vi "SaveWWWImages2.vi"(7 "Tab charts":refnum<vi>, 9 "Image Data 2":T1, 10 "Destination":path, 11 "VI in":refnum<vi>) -> ()   [LabVIEW 2017]
uses:
  Web Imge control.ctl
panel:
  out "Write Imegtime":u32
  out "get Imegtime":u32
  out "Time":u32
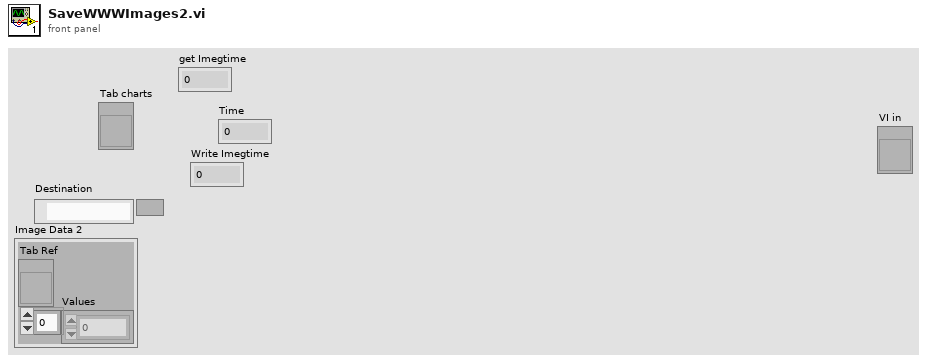
[diagram p1: front panel]
types:
  T1 = typedef "Web Imge control.ctl" = cluster{"Tab Ref":refnum<vi>, "Values":i32[]}
  T2 = typedef "imagedata.ctl" = cluster{"image type":i32, "image depth":i32, "image":u8[], "mask":u8[], "colors":u32[], "Rectangle":cluster{"left":i16, "top":i16, "right":i16, "bottom":i16}}
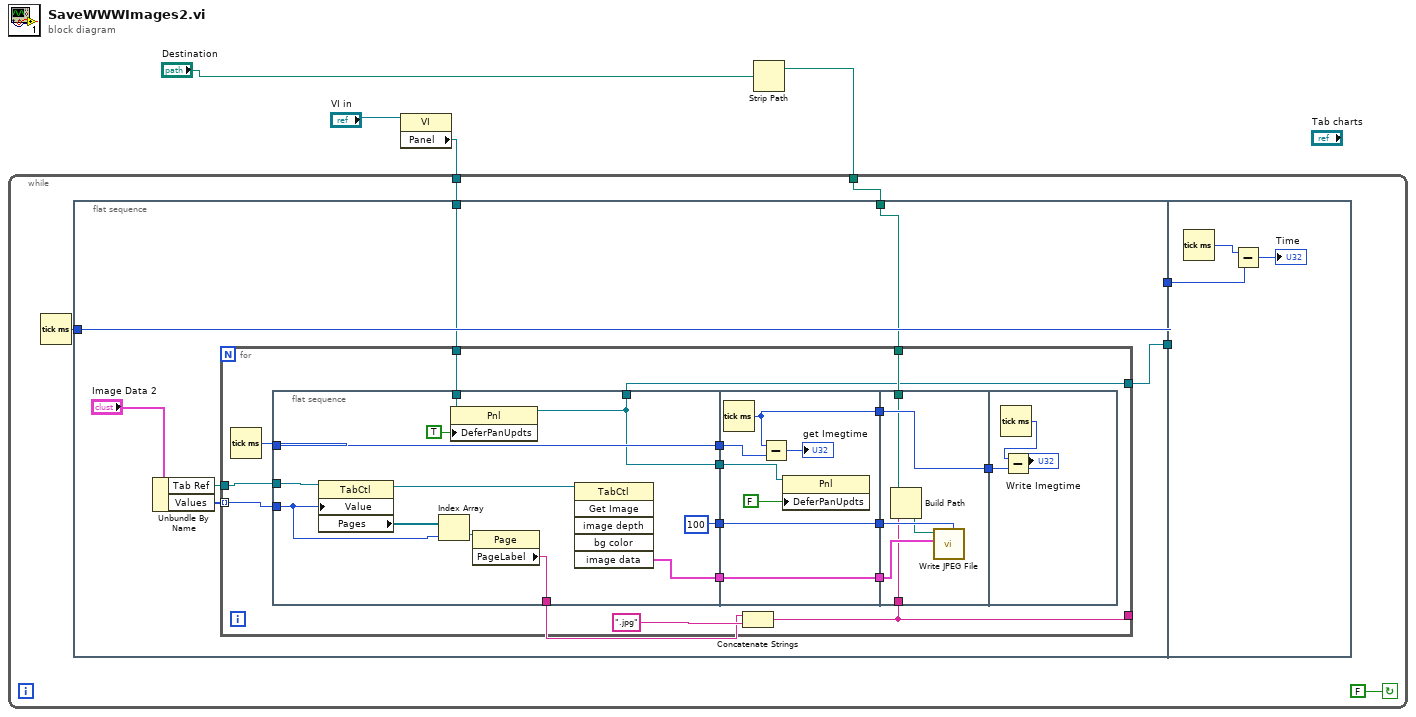
[diagram p0: block diagram]
diagram:
  n1 = property class="VI"(reference="VI in") -> ("Panel"=w1:refnum<vi>)  [unwired: 1 in, 2 out]
  n2 = Strip Path(path="Destination") -> (stripped path=w2:path)  [unwired: 1 out]
  n3 = while {
    tunnel: w2 -> [w6]
    tunnel: w1 -> [w5]
    stop <- FALSE continue-if-true
    n4 = Tick Count (ms)() -> (millisecond timer value=w8:u32)
    n5 = flat-sequence {
      tunnel: [w11] -> w10
      tunnel: [w17] -> w9
      tunnel: w8 -> [w17]
      tunnel: w6 -> [w13]
      tunnel: w5 -> [w12]
      tunnel: w10 -> [_]
      tunnel: w9 -> [w64]
      frame #0 {
        n6 = Unbundle By Name("Image Data 2") -> ("Tab Ref"=w16:refnum<vi>, "Values"=w15:i32[])
        n7 = for {
          tunnel: [w21] -> _
          tunnel: w16 -> [w25]
          tunnel: w15 -> [w24] mode=indexing
          tunnel: w13 -> [w22]
          tunnel: w12 -> [w20]
          tunnel: [w19] -> w11
          n8 = Tick Count (ms)() -> (millisecond timer value=w26:u32)
          n9 = flat-sequence {
            tunnel: w25 -> [w46]
            tunnel: [w44] -> w34
            tunnel: [100 ("quality (80)")] -> w33
            tunnel: [w42] -> w32
            tunnel: w26 -> [w42]
            tunnel: w24 -> [w41]
            tunnel: [w38] -> w23
            tunnel: w20 -> [w37]
            tunnel: [w35] -> w19
            tunnel: [w35] -> w18
            tunnel: w34 -> [w53]
            tunnel: [w53] -> w31
            tunnel: w33 -> [w52]
            tunnel: [w52] -> w30
            tunnel: w32 -> [w51]
            tunnel: [w49] -> w29
            tunnel: w18 -> [w47]
            tunnel: w31 -> [w58]
            tunnel: w30 -> [w59]
            tunnel: w29 -> [w57]
            tunnel: [w57] -> w28
            tunnel: w22 -> [w56]
            tunnel: w21 -> [w54]
            tunnel: w28 -> [w60]
            frame #0 {
              n10 = property class="TabCtl"(reference=w46, "Value"=w41) -> (reference out=w45:refnum<vi>, "Pages"=w40:refnum<vi>[])  [unwired: 1 in, 1 out]
              n11 = Index Array(array=w40, index=w41) -> (element=w39:refnum<vi>)
              n12 = property class="Pnl"(reference=w37, "DeferPanUpdts"=TRUE ("Defer Panel Updates")) -> (reference out=w35:refnum<vi>)  [unwired: 1 in, 1 out]
              n13 = property class="Page"(reference=w39) -> ("PageLabel"=w38:string)  [unwired: 1 in, 2 out]
              n14 = invoke class="TabCtl" method="Get Image"(reference=w45) -> ("image data"=w44:T2)  [unwired: 5 in, 5 out]
            }
            frame #1 {
              n15 = Tick Count (ms)() -> (millisecond timer value=w49:u32)
              n16 = Subtract(x=w49, y=w51) -> (x-y=→"get Imegtime":u32)
              n17 = property class="Pnl"(reference=w47, "DeferPanUpdts"=FALSE ("Defer Panel Updates")) -> ()  [unwired: 1 in, 2 out]
            }
            frame #2 {
              n18 = Build Path(base path=w56, name or relative path=w54) -> (appended path=w55:path)
              n19 = call <vilib>:"Write JPEG File.vi"("quality (80)"=w59, "image data"=w58, "path to JPEG file"=w55) -> ()  [unwired: 7 in, 2 out]
            }
            frame #3 {
              n20 = Tick Count (ms)() -> (millisecond timer value=w61:u32)
              n21 = Subtract(x=w61, y=w60) -> (x-y=→"Write Imegtime":u32)
            }
          }
          n22 = Concatenate Strings(w23, ".jpg" ("string")) -> (w21:string)
        }
      }
      frame #1 {
        n23 = Tick Count (ms)() -> (millisecond timer value=w65:u32)
        n24 = Subtract(x=w65, y=w64) -> (x-y=→"Time":u32)
      }
    }
  }
